vi "ExecuteSequentialOperations.vi"(4 "Item Names":string[](array[string]), 5 "threshold":cluster{u8, u8}, 6 "Plane In":T1 {"Dialogs" format="%.0b"}) -> (1 "8 Bit out":T1 {"Dialogs" format="%.0b"}, 2 "Image Out":T1 {"Dialogs" format="%.0b"})   [LabVIEW 2010]
uses:
  <userlib>/ImageProcessing/QTLIB_2595_LV86/QT_Image.ctl
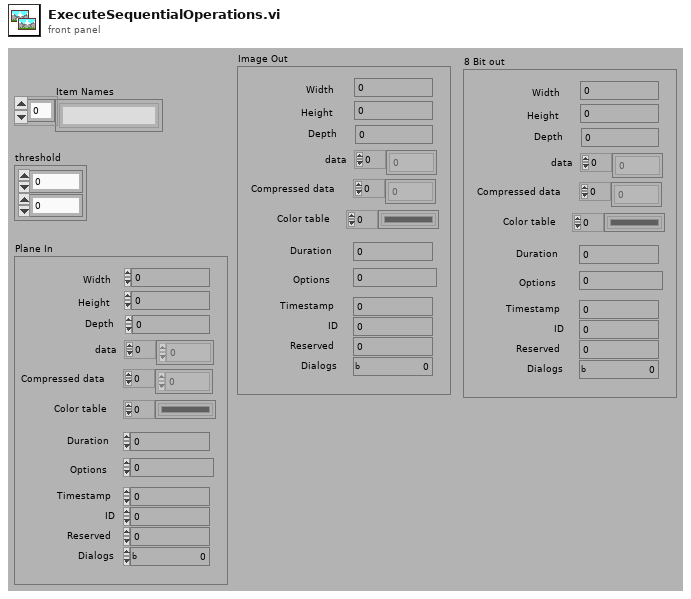
[diagram p1: front panel]
types:
  T1 = typedef "QT_Image.ctl" = cluster{"Width":i32, "Height":i32, "Depth":i32, "data":u8[], "Compressed data":u8[], "Color table":u32[], "Duration":i32, "Options":i32, "Timestamp":i32, "ID":i32, "Reserved":i32, "Dialogs":u32}
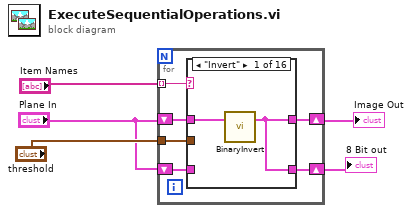
[diagram p0: block diagram]
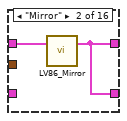
[diagram p2: hidden frame]
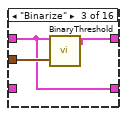
[diagram p3: hidden frame]
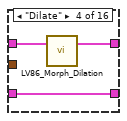
[diagram p4: hidden frame]
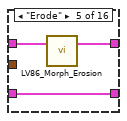
[diagram p5: hidden frame]
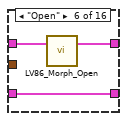
[diagram p6: hidden frame]
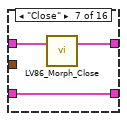
[diagram p7: hidden frame]
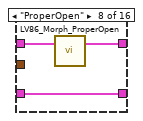
[diagram p8: hidden frame]
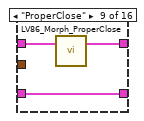
[diagram p9: hidden frame]
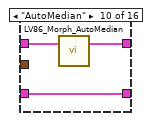
[diagram p10: hidden frame]
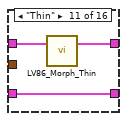
[diagram p11: hidden frame]
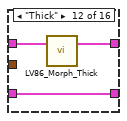
[diagram p12: hidden frame]
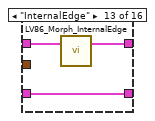
[diagram p13: hidden frame]
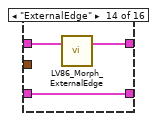
[diagram p14: hidden frame]
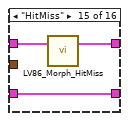
[diagram p15: hidden frame]
diagram:
  n1 = for {
    shift-right: [w10] -> w4
    shift-left: "Plane In" -> [w9]
    tunnel: "Item Names" -> [w11] mode=indexing
    tunnel: "threshold" -> [w8]
    shift-right: [w7] -> w1
    shift-left: "Plane In" -> [w6]
    n2 = case shown="\"Invert\"" w11 {
      tunnel: [w12 w14 w18 w20 w23 w26 w29 w32 w35 w38 w41 w44 w47 w50 w53 w56] -> w10
      tunnel: w9 -> [w13 w15 w16 w21 w24 w27 w30 w33 w36 w39 w42 w45 w48 w51 w54 w56]
      tunnel: w8 -> [_ _ w17 _ _ _ _ _ _ _ _ _ _ _ _ _]
      tunnel: [w12 w14 w16 w19 w22 w25 w28 w31 w34 w37 w40 w43 w46 w49 w52 w55] -> w7
      tunnel: w6 -> [_ _ _ w19 w22 w25 w28 w31 w34 w37 w40 w43 w46 w49 w52 w55]
      frame "Invert" {
        n3 = call <userlib>:"BinaryInvert.vi"("Image In"=w13) -> ("Image Out"=w12:T1)  [unwired: 2 in]
      }
      frame "Mirror" {
        n4 = call <userlib>:"LV86_Mirror.vi"("Image"=w15) -> ("Image"=w14:T1)  [unwired: 2 in]
      }
      frame "Binarize" {
        n5 = call <userlib>:"BinaryThreshold.vi"("threshold"=w17, "Image In"=w16) -> ("Image Out"=w18:T1)  [unwired: 1 in]
      }
      frame "Dilate" {
        n6 = call <userlib>:"LV86_Morph_Dilation.vi"("Image in"=w21) -> ("Image out"=w20:T1)  [unwired: 2 in]
      }
      frame "Erode" {
        n7 = call <userlib>:"LV86_Morph_Erosion.vi"("Image in"=w24) -> ("Image out"=w23:T1)  [unwired: 2 in]
      }
      frame "Open" {
        n8 = call <userlib>:"LV86_Morph_Open.vi"("Image in"=w27) -> ("Image out"=w26:T1)  [unwired: 2 in]
      }
      frame "Close" {
        n9 = call <userlib>:"LV86_Morph_Close.vi"("Image in"=w30) -> ("Image out"=w29:T1)  [unwired: 2 in]
      }
      frame "ProperOpen" {
        n10 = call <userlib>:"LV86_Morph_ProperOpen.vi"("Image in"=w33) -> ("Image out"=w32:T1)  [unwired: 2 in]
      }
      frame "ProperClose" {
        n11 = call <userlib>:"LV86_Morph_ProperClose.vi"("Image in"=w36) -> ("Image out"=w35:T1)  [unwired: 2 in]
      }
      frame "AutoMedian" {
        n12 = call <userlib>:"LV86_Morph_AutoMedian.vi"("Image in"=w39) -> ("Image out"=w38:T1)  [unwired: 2 in]
      }
      frame "Thin" {
        n13 = call <userlib>:"LV86_Morph_Thin.vi"("Image in"=w42) -> ("Image out"=w41:T1)  [unwired: 2 in]
      }
      frame "Thick" {
        n14 = call <userlib>:"LV86_Morph_Thick.vi"("Image in"=w45) -> ("Image out"=w44:T1)  [unwired: 2 in]
      }
      frame "InternalEdge" {
        n15 = call <userlib>:"LV86_Morph_InternalEdge.vi"("Image in"=w48) -> ("Image out"=w47:T1)  [unwired: 2 in]
      }
      frame "ExternalEdge" {
        n16 = call <userlib>:"LV86_Morph_ExternalEdge.vi"("Image in"=w51) -> ("Image out"=w50:T1)  [unwired: 2 in]
      }
      frame "HitMiss" {
        n17 = call <userlib>:"LV86_Morph_HitMiss.vi"("Image in"=w54) -> ("Image out"=w53:T1)  [unwired: 2 in]
      }
      frame Default {
      }
    }
  }
  "Image Out" <- w4
  "8 Bit out" <- w1
